vi "write_T.vi"(7 "Enum":T1(ring), 8 "error in":errorcluster, 9 "Data":dbl, 10 "physical channels":tag) -> (0 "error out":errorcluster)   [LabVIEW 2015]
uses:
  <vilib>/DAQmx/write.llb/DAQmx Write (Analog DBL 1Chan 1Samp).vi
  <vilib>/DAQmx/create/channels.llb/DAQmx Create Channel (AO-Voltage-Basic).vi
  <vilib>/DAQmx/miscellaneous.llb/DAQmx Fill In Error Info.vi
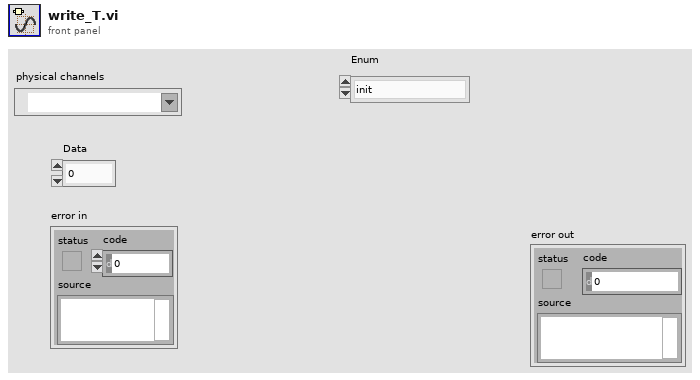
[diagram p1: front panel]
types:
  T1 = enum16{"init", "config", "start", "write", "stop"}
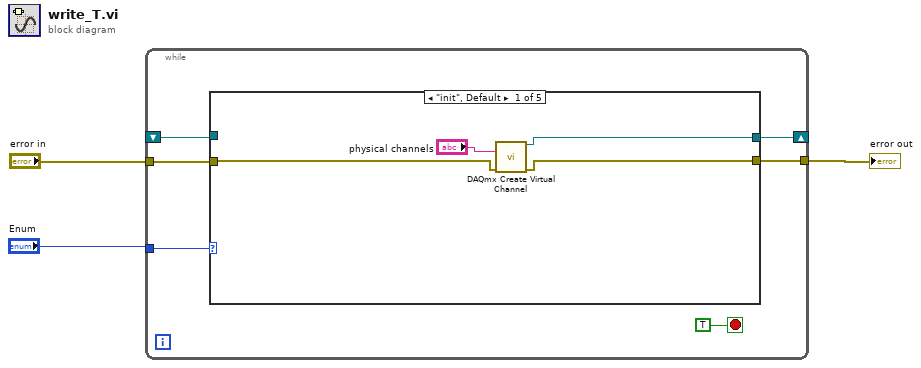
[diagram p0: block diagram]
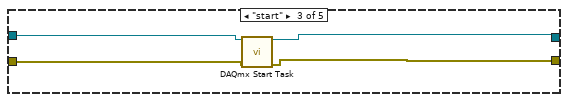
[diagram p3: hidden frame]
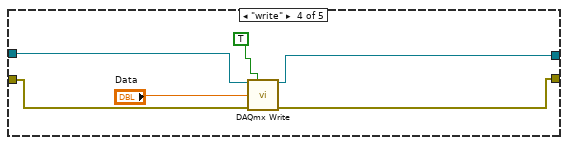
[diagram p4: hidden frame]
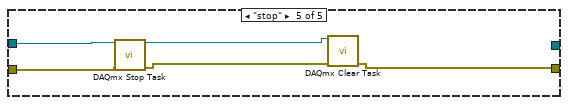
[diagram p5: hidden frame]
diagram:
  n1 = while {
    tunnel: "Enum" -> [w8]
    shift-right: [w7] -> _
    shift-left: _ -> [w6]
    tunnel: "error in" -> [w5]
    tunnel: [w4] -> w1
    stop <- TRUE stop-if-true
    n2 = case shown="\"init\", Default" w8 {
      tunnel: [w11 w15 w18 w23 _] -> w7
      tunnel: w6 -> [_ w15 w19 w25 w30]
      tunnel: w5 -> [w13 w14 w17 w22 w29]
      tunnel: [w12 w14 w16 w21 w28] -> w4
      frame "init", Default {
        n3 = call-poly <vilib>:"DAQmx Create Virtual Channel.vi"("physical channels"="physical channels", "error in"=w13) -> ("task out"=w11:refnum<k21>, "error out"=w12:errorcluster)  [unwired: 12 in]
      }
      frame "config" {
      }
      frame "start" {
        n4 = call <vilib>:"DAQmx Start Task.vi"("task/channels in"=w19, "error in"=w17) -> ("task out"=w18:refnum<k21>, "error out"=w16:errorcluster)  [unwired: 12 in]
      }
      frame "write" {
        n5 = call-poly <vilib>:"DAQmx Write.vi"("task/channels in"=w25, "auto start"=TRUE, "data"="Data", "error in"=w22) -> ("task out"=w23:refnum<k21>, "error out"=w21:errorcluster)  [unwired: 9 in, 1 out]
      }
      frame "stop" {
        n6 = call <vilib>:"DAQmx Stop Task.vi"("task/channels in"=w30, "error in"=w29) -> ("task out"=w27:refnum<k21>, "error out"=w26:errorcluster)  [unwired: 12 in]
        n7 = call <vilib>:"DAQmx Clear Task.vi"("task in"=w27, "error in"=w26) -> ("error out"=w28:errorcluster)  [unwired: 13 in]
      }
    }
  }
  "error out" <- w1
